vi "Junkie.vi"() -> ()   [LabVIEW 2016]
panel:
  out "x/y":dbl
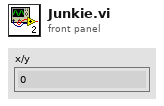
[diagram p1: front panel]
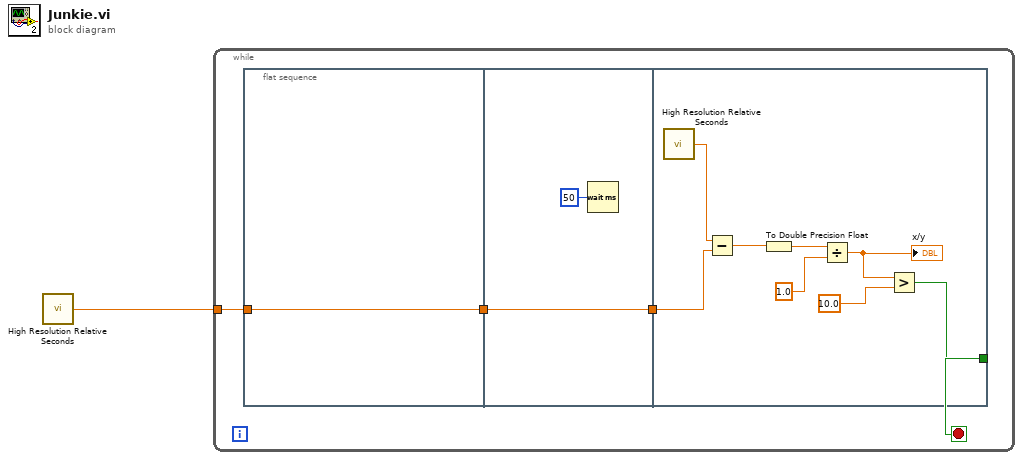
[diagram p0: block diagram]
diagram:
  n1 = call <vilib>:"High Resolution Relative Seconds.vi"() -> ("relative seconds"=w1:dbl)
  n2 = while {
    tunnel: w1 -> [w4]
    stop <- w5 stop-if-true
    n3 = flat-sequence {
      tunnel: w4 -> [w6]
      tunnel: [w6] -> w3
      tunnel: w3 -> [w8]
      tunnel: [w8] -> w2
      tunnel: [w11] -> w5
      tunnel: w2 -> [w9]
      frame #0 {
      }
      frame #1 {
        n4 = Wait (ms)(milliseconds to wait=u32 50) -> ()  [unwired: 1 out]
      }
      frame #2 {
        n5 = call <vilib>:"High Resolution Relative Seconds.vi"() -> ("relative seconds"=w10:dbl)
        n6 = Subtract(x=w10, y=w9) -> (x-y=w16:dbl)
        n7 = To Double Precision Float(number=w16) -> (double precision float=w15:dbl)
        n8 = Divide(x=w15, y=1.0) -> (x/y=w13:dbl)
        "x/y" <- w13
        n9 = Greater?(x=w13, y=10.0) -> (0:w11:bool)
      }
    }
  }
